vi "FPGA Values View.vi"() -> ()   [LabVIEW 2016, in "M1M3SupportEUI_Views.lvlib"]
uses:
  M1M3SupportEUI_Views.lvlib
  Model/Model.lvclass
  M1M3 Support Events/M1M3 Support Events.lvclass/M1M3 Support Events.ctl
  Typedefs/StateTypes.ctl
  M1M3 Support Events/M1M3 Support Events.lvclass
  Typedefs/M1M3SupportEUI_TypeDefs.lvlib
panel:
  out "Slewing?":string
  out "BroadcastCounter":u8
  out "OuterLoop Time Stamp":timestamp
  out "MRFC 5":u32
  out "MRFC 4":u32
  out "MRFC 3":u32
  out "MRFC 2":u32
  out "MRFC 1":u32
  out "MRBC 5":u32
  out "MRBC 4":u32
  out "MRBC 3":u32
  out "MRBC 2":u32
  out "MRBC 1":u32
  out "MTFC 5":u32
  out "MTFC 4":u32
  out "MTFC 3":u32
  out "MTFC 2":u32
  out "MTFC 1":u32
  out "MTBC 5":u32
  out "MTBC 4":u32
  out "MTBC 3":u32
  out "MTBC 2":u32
  out "MTBC 1":u32
  out "MRDFO 5":string
  out "MRDFO 4":string
  out "MRDFO 3":string
  out "MRDFO 2":string
  out "MRDFO 1":string
  out "MStpBE 5":string
  out "MStpBE 4":string
  out "MStpBE 3":string
  out "MStpBE 2":string
  out "MStpBE 1":string
  out "MStrtBE 5":string
  out "MStrtBE 4":string
  out "MStrtBE 3":string
  out "MStrtBE 2":string
  out "MStrtBE 1":string
  out "MWFRT 5":string
  out "MWFRT 4":string
  out "MWFRT 3":string
  out "MWFRT 2":string
  out "MWFRT 1":string
  out "MII 5":string
  out "MII 4":string
  out "MII 3":string
  out "MII 2":string
  out "MII 1":string
  out "MTIFO1 5":string
  out "MTIFO1 4":string
  out "MTIFO1 3":string
  out "MTIFO1 2":string
  out "MTIFO1":string
  out "FPGA Time Stamp":timestamp
  out "SAL Time Stamp":timestamp
  in  "Model in":refnum<class "Model.lvclass">
  # "FPGA/Outer Loop Data Values"
  # "FPGA"
  # "1"
  # "2"
  # "3"
  # "4"
  # "5"
  # "Modbus TX Internal FIFO Overflow"
  # "Modbus Invalid Instruction"
  # "Modbus Wait For RX Frame Timeout"
  # "Modbus Start Bit Error"
  # "Modbus Stop Bit Error"
  # "Modbus RX Data FIFO Overflow"
  # "Modbus TX Byte Count"
  # "Modbus Tx Frame Count"
  # "Modbus Rx Byte Count"
  # "Modbus Rx Frame Count"
  # "Outer Loop"
  # "Broadcast counter"
  # "Slewing?"
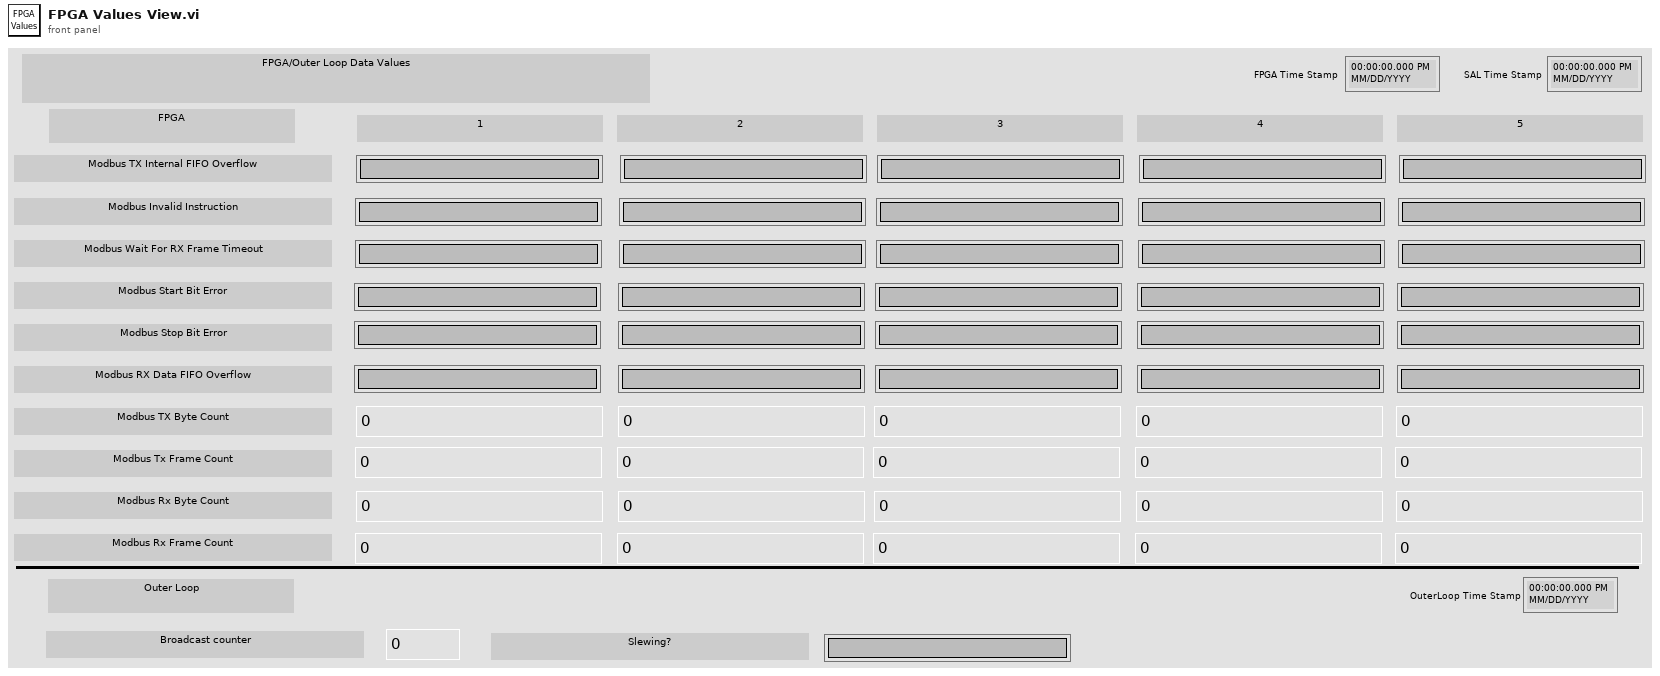
[diagram p1: front panel]
types:
  T1 = typedef "M1M3SupportEUI_TypeDefs.lvlib/M1M3 Support Events.ctl" = cluster{"M1M3 Support State":refnum<user-event>, "Inclinometer  Data":refnum<user-event>, "IMS Data":refnum<user-event>, "FA Data":refnum<user-event>, "FA Status":refnum<user-event>, "SAL Connected":refnum<user-event>, "HP Data":refnum<user-event>, "HP Status":refnum<user-event>, "Accelerometer Data":refnum<user-event>, "FPGA Data":refnum<user-event>, "Inclinometer Data":refnum<user-event>, "MirrorForces Data":refnum<user-event>, "OuterLoop Data":refnum<user-event>, "ErrorCode Event":refnum<user-event>, "InterlockStatus Event":refnum<user-event>, "InterlockWarning Event":refnum<user-event>}
  T2 = typedef "M1M3SupportEUI_TypeDefs.lvlib/StateTypes.ctl" = u32
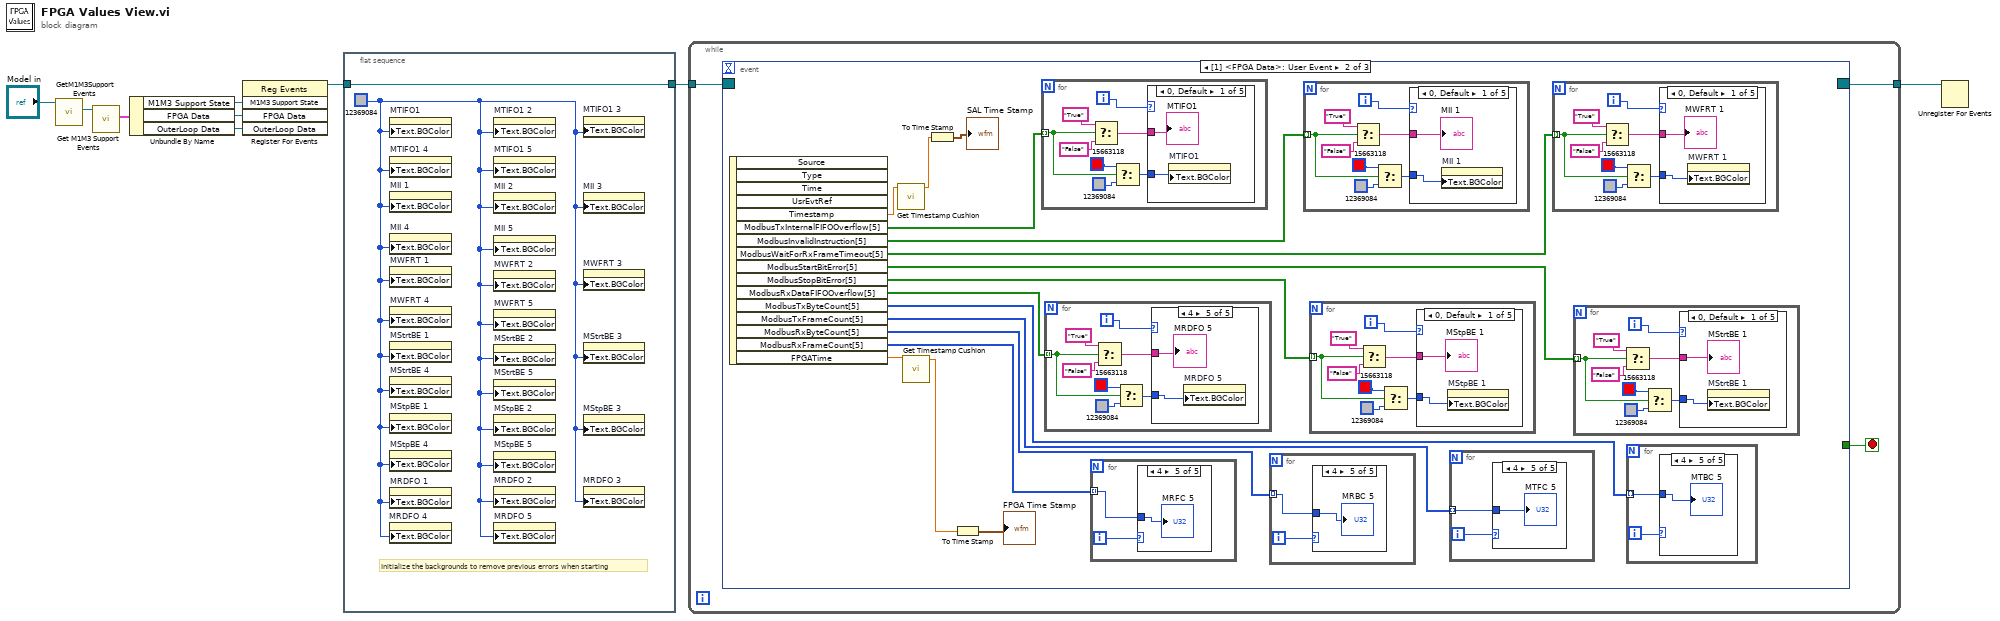
[diagram p0: block diagram]
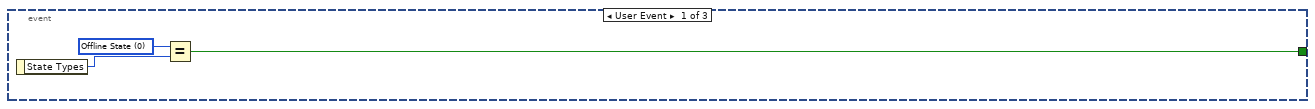
[diagram p2: hidden frame]
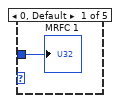
[diagram p3: hidden frame]
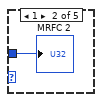
[diagram p4: hidden frame]
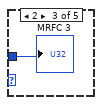
[diagram p5: hidden frame]
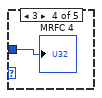
[diagram p6: hidden frame]
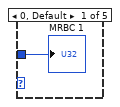
[diagram p7: hidden frame]
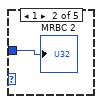
[diagram p8: hidden frame]
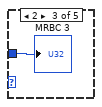
[diagram p9: hidden frame]
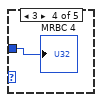
[diagram p10: hidden frame]
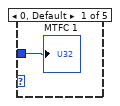
[diagram p11: hidden frame]
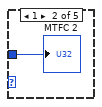
[diagram p12: hidden frame]
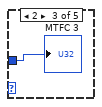
[diagram p13: hidden frame]
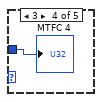
[diagram p14: hidden frame]
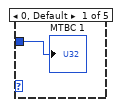
[diagram p15: hidden frame]
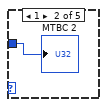
[diagram p16: hidden frame]
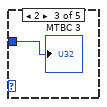
[diagram p17: hidden frame]
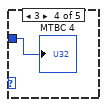
[diagram p18: hidden frame]
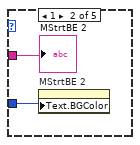
[diagram p19: hidden frame]
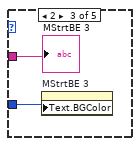
[diagram p20: hidden frame]
diagram:
  n1 = call "GetM1M3SupportEvents.vi"("Model in"="Model in") -> ("M1M3 Support Events out"=w5:refnum<class "M1M3 Support Events.lvclass">)  [unwired: 8 in, 2 out]
  n2 = call "Get M1M3 Support Events.vi"("M1M3 Support Events in"=w5) -> ("M1M3 Support Events"=w6:T1)  [unwired: 9 in, 1 out]
  n3 = Unbundle By Name(w6) -> ("M1M3 Support State"=w8:refnum<user-event>, "FPGA Data"=w9:refnum<user-event>, "OuterLoop Data"=w3:refnum<user-event>)
  n4 = register-events(w8, w9, w3) -> (reference out=w2:refnum<event-registration>)  [unwired: 2 in, 1 out]
  n5 = flat-sequence {
    tunnel: w2 -> [w10]
    tunnel: [w10] -> w1
    frame #0 {
      w11 = u32 12369084
      # "Initialize the backgrounds to remove previous errors when starting"
      n6 = property on="MTIFO1" class="Str"("Text.BGColor"=w11) -> ()  [unwired: 2 in, 2 out]
      n7 = property on="MTIFO1 4" class="Str"("Text.BGColor"=w11) -> ()  [unwired: 2 in, 2 out]
      n8 = property on="MII 1" class="Str"("Text.BGColor"=w11) -> ()  [unwired: 2 in, 2 out]
      n9 = property on="MII 4" class="Str"("Text.BGColor"=w11) -> ()  [unwired: 2 in, 2 out]
      n10 = property on="MWFRT 1" class="Str"("Text.BGColor"=w11) -> ()  [unwired: 2 in, 2 out]
      n11 = property on="MWFRT 4" class="Str"("Text.BGColor"=w11) -> ()  [unwired: 2 in, 2 out]
      n12 = property on="MStrtBE 1" class="Str"("Text.BGColor"=w11) -> ()  [unwired: 2 in, 2 out]
      n13 = property on="MStrtBE 4" class="Str"("Text.BGColor"=w11) -> ()  [unwired: 2 in, 2 out]
      n14 = property on="MStpBE 1" class="Str"("Text.BGColor"=w11) -> ()  [unwired: 2 in, 2 out]
      n15 = property on="MStpBE 4" class="Str"("Text.BGColor"=w11) -> ()  [unwired: 2 in, 2 out]
      n16 = property on="MRDFO 1" class="Str"("Text.BGColor"=w11) -> ()  [unwired: 2 in, 2 out]
      n17 = property on="MRDFO 4" class="Str"("Text.BGColor"=w11) -> ()  [unwired: 2 in, 2 out]
      n18 = property on="MTIFO1 2" class="Str"("Text.BGColor"=w11) -> ()  [unwired: 2 in, 2 out]
      n19 = property on="MTIFO1 5" class="Str"("Text.BGColor"=w11) -> ()  [unwired: 2 in, 2 out]
      n20 = property on="MII 2" class="Str"("Text.BGColor"=w11) -> ()  [unwired: 2 in, 2 out]
      n21 = property on="MII 5" class="Str"("Text.BGColor"=w11) -> ()  [unwired: 2 in, 2 out]
      n22 = property on="MWFRT 2" class="Str"("Text.BGColor"=w11) -> ()  [unwired: 2 in, 2 out]
      n23 = property on="MWFRT 5" class="Str"("Text.BGColor"=w11) -> ()  [unwired: 2 in, 2 out]
      n24 = property on="MStrtBE 2" class="Str"("Text.BGColor"=w11) -> ()  [unwired: 2 in, 2 out]
      n25 = property on="MStrtBE 5" class="Str"("Text.BGColor"=w11) -> ()  [unwired: 2 in, 2 out]
      n26 = property on="MStpBE 2" class="Str"("Text.BGColor"=w11) -> ()  [unwired: 2 in, 2 out]
      n27 = property on="MStpBE 5" class="Str"("Text.BGColor"=w11) -> ()  [unwired: 2 in, 2 out]
      n28 = property on="MRDFO 2" class="Str"("Text.BGColor"=w11) -> ()  [unwired: 2 in, 2 out]
      n29 = property on="MRDFO 5" class="Str"("Text.BGColor"=w11) -> ()  [unwired: 2 in, 2 out]
      n30 = property on="MTIFO1 3" class="Str"("Text.BGColor"=w11) -> ()  [unwired: 2 in, 2 out]
      n31 = property on="MII 3" class="Str"("Text.BGColor"=w11) -> ()  [unwired: 2 in, 2 out]
      n32 = property on="MWFRT 3" class="Str"("Text.BGColor"=w11) -> ()  [unwired: 2 in, 2 out]
      n33 = property on="MStrtBE 3" class="Str"("Text.BGColor"=w11) -> ()  [unwired: 2 in, 2 out]
      n34 = property on="MStpBE 3" class="Str"("Text.BGColor"=w11) -> ()  [unwired: 2 in, 2 out]
      n35 = property on="MRDFO 3" class="Str"("Text.BGColor"=w11) -> ()  [unwired: 2 in, 2 out]
    }
  }
  n36 = while {
    tunnel: w1 -> [w14]
    tunnel: [w12] -> w4
    stop <- w13 stop-if-true
    n37 = event shown="[1] <FPGA Data>: User Event" {
      selector: w14 -> [_ _ _]
      dyn-events: [_ _ _] -> w12
      timeout: _ -> [_ _ _]
      tunnel: [w15 _ _] -> w13
      event User Event {
        w16 = T2 0 items=["Offline State"=0, "Fault State"=4294967295, "Standby State"=16777216, "Disabled State"=33554432, "Enabled State"=50331648, "Parked State"=50331649, "Raising State"=50331650, "Active State"=50331651, "Lowering State"=50331652, "Engineering State"=50397184, "Parked Engineering State"=50397185, "Raising Engineering State"=50397186, "Active Engineering State"=50397187, "Lowering Engineering State"=50397188] ("x")
        n38 = event-data() -> ("State Types"=w17:T2)  [unwired: 1 in]
        n39 = Equal?(x=w16, y=w17) -> (x = y?=w15:bool)
      }
      event User Event {
        n40 = event-data() -> ("Timestamp"=w19:dbl, "ModbusTxInternalFIFOOverflow[5]"=w33:bool[], "ModbusInvalidInstruction[5]"=w32:bool[], "ModbusWaitForRxFrameTimeout[5]"=w31:bool[], "ModbusStartBitError[5]"=w28:bool[], "ModbusStopBitError[5]"=w29:bool[], "ModbusRxDataFIFOOverflow[5]"=w30:bool[], "ModbusTxByteCount[5]"=w27:u32[], "ModbusTxFrameCount[5]"=w26:u32[], "ModbusRxByteCount[5]"=w25:u32[], "ModbusRxFrameCount[5]"=w24:u32[], "FPGATime"=w21:dbl)  [unwired: 1 in, 4 out]
        n41 = call "Get Timestamp Cushion.vi"("DoubleTimestampRepresentation"=w19) -> ("TimestampCushion"=w18:dbl)  [unwired: 10 in]
        n42 = call "Get Timestamp Cushion.vi"("DoubleTimestampRepresentation"=w21) -> ("TimestampCushion"=w20:dbl)  [unwired: 10 in]
        n43 = To Time Stamp(1:w18) -> (0:→"SAL Time Stamp":timestamp)
        n44 = To Time Stamp(1:w20) -> (0:→"FPGA Time Stamp":timestamp)
        n45 = for {
          tunnel: w33 -> [w153] mode=indexing
          i -> [w157]
          n46 = Select(t="True", s=w153, f="False") -> (s? t:f=w156:string)
          n47 = Select(t=u32 15663118, s=w153, f=u32 12369084) -> (s? t:f=w152:u32)
          n48 = case shown="0, Default" w157 {
            tunnel: w156 -> [w161 w163 w165 w167 w169]
            tunnel: w152 -> [w160 w162 w164 w166 w168]
            frame 0, Default {
              n49 = property on="MTIFO1" class="Str"("Text.BGColor"=w160) -> ()  [unwired: 2 in, 2 out]
              "MTIFO1" <- w161
            }
            frame 1 {
              n50 = property on="MTIFO1 2" class="Str"("Text.BGColor"=w162) -> ()  [unwired: 2 in, 2 out]
              "MTIFO1 2" <- w163
            }
            frame 2 {
              n51 = property on="MTIFO1 3" class="Str"("Text.BGColor"=w164) -> ()  [unwired: 2 in, 2 out]
              "MTIFO1 3" <- w165
            }
            frame 3 {
              n52 = property on="MTIFO1 4" class="Str"("Text.BGColor"=w166) -> ()  [unwired: 2 in, 2 out]
              "MTIFO1 4" <- w167
            }
            frame 4 {
              n53 = property on="MTIFO1 5" class="Str"("Text.BGColor"=w168) -> ()  [unwired: 2 in, 2 out]
              "MTIFO1 5" <- w169
            }
          }
        }
        n54 = for {
          tunnel: w30 -> [w99] mode=indexing
          i -> [w103]
          n55 = Select(t="True", s=w99, f="False") -> (s? t:f=w102:string)
          n56 = Select(t=u32 15663118, s=w99, f=u32 12369084) -> (s? t:f=w98:u32)
          n57 = case shown="4" w103 {
            tunnel: w102 -> [w107 w109 w111 w113 w115]
            tunnel: w98 -> [w106 w108 w110 w112 w114]
            frame 0, Default {
              n58 = property on="MRDFO 1" class="Str"("Text.BGColor"=w106) -> ()  [unwired: 2 in, 2 out]
              "MRDFO 1" <- w107
            }
            frame 1 {
              n59 = property on="MRDFO 2" class="Str"("Text.BGColor"=w108) -> ()  [unwired: 2 in, 2 out]
              "MRDFO 2" <- w109
            }
            frame 2 {
              n60 = property on="MRDFO 3" class="Str"("Text.BGColor"=w110) -> ()  [unwired: 2 in, 2 out]
              "MRDFO 3" <- w111
            }
            frame 3 {
              n61 = property on="MRDFO 4" class="Str"("Text.BGColor"=w112) -> ()  [unwired: 2 in, 2 out]
              "MRDFO 4" <- w113
            }
            frame 4 {
              n62 = property on="MRDFO 5" class="Str"("Text.BGColor"=w114) -> ()  [unwired: 2 in, 2 out]
              "MRDFO 5" <- w115
            }
          }
        }
        n63 = for {
          tunnel: w24 -> [w34] mode=indexing
          i -> [w35]
          n64 = case shown="4" w35 {
            tunnel: w34 -> [w36 w37 w38 w39 w40]
            frame 0, Default {
              "MRFC 1" <- w36
            }
            frame 1 {
              "MRFC 2" <- w37
            }
            frame 2 {
              "MRFC 3" <- w38
            }
            frame 3 {
              "MRFC 4" <- w39
            }
            frame 4 {
              "MRFC 5" <- w40
            }
          }
        }
        n65 = for {
          tunnel: w25 -> [w41] mode=indexing
          i -> [w42]
          n66 = case shown="4" w42 {
            tunnel: w41 -> [w43 w44 w45 w46 w47]
            frame 0, Default {
              "MRBC 1" <- w43
            }
            frame 1 {
              "MRBC 2" <- w44
            }
            frame 2 {
              "MRBC 3" <- w45
            }
            frame 3 {
              "MRBC 4" <- w46
            }
            frame 4 {
              "MRBC 5" <- w47
            }
          }
        }
        n67 = for {
          tunnel: w32 -> [w135] mode=indexing
          i -> [w139]
          n68 = Select(t="True", s=w135, f="False") -> (s? t:f=w138:string)
          n69 = Select(t=u32 15663118, s=w135, f=u32 12369084) -> (s? t:f=w134:u32)
          n70 = case shown="0, Default" w139 {
            tunnel: w138 -> [w143 w145 w147 w149 w151]
            tunnel: w134 -> [w142 w144 w146 w148 w150]
            frame 0, Default {
              n71 = property on="MII 1" class="Str"("Text.BGColor"=w142) -> ()  [unwired: 2 in, 2 out]
              "MII 1" <- w143
            }
            frame 1 {
              n72 = property on="MII 2" class="Str"("Text.BGColor"=w144) -> ()  [unwired: 2 in, 2 out]
              "MII 2" <- w145
            }
            frame 2 {
              n73 = property on="MII 3" class="Str"("Text.BGColor"=w146) -> ()  [unwired: 2 in, 2 out]
              "MII 3" <- w147
            }
            frame 3 {
              n74 = property on="MII 4" class="Str"("Text.BGColor"=w148) -> ()  [unwired: 2 in, 2 out]
              "MII 4" <- w149
            }
            frame 4 {
              n75 = property on="MII 5" class="Str"("Text.BGColor"=w150) -> ()  [unwired: 2 in, 2 out]
              "MII 5" <- w151
            }
          }
        }
        n76 = for {
          tunnel: w29 -> [w81] mode=indexing
          i -> [w85]
          n77 = Select(t="True", s=w81, f="False") -> (s? t:f=w84:string)
          n78 = Select(t=u32 15663118, s=w81, f=u32 12369084) -> (s? t:f=w80:u32)
          n79 = case shown="0, Default" w85 {
            tunnel: w84 -> [w89 w91 w93 w95 w97]
            tunnel: w80 -> [w88 w90 w92 w94 w96]
            frame 0, Default {
              n80 = property on="MStpBE 1" class="Str"("Text.BGColor"=w88) -> ()  [unwired: 2 in, 2 out]
              "MStpBE 1" <- w89
            }
            frame 1 {
              n81 = property on="MStpBE 2" class="Str"("Text.BGColor"=w90) -> ()  [unwired: 2 in, 2 out]
              "MStpBE 2" <- w91
            }
            frame 2 {
              n82 = property on="MStpBE 3" class="Str"("Text.BGColor"=w92) -> ()  [unwired: 2 in, 2 out]
              "MStpBE 3" <- w93
            }
            frame 3 {
              n83 = property on="MStpBE 4" class="Str"("Text.BGColor"=w94) -> ()  [unwired: 2 in, 2 out]
              "MStpBE 4" <- w95
            }
            frame 4 {
              n84 = property on="MStpBE 5" class="Str"("Text.BGColor"=w96) -> ()  [unwired: 2 in, 2 out]
              "MStpBE 5" <- w97
            }
          }
        }
        n85 = for {
          tunnel: w26 -> [w48] mode=indexing
          i -> [w49]
          n86 = case shown="4" w49 {
            tunnel: w48 -> [w50 w51 w52 w53 w54]
            frame 0, Default {
              "MTFC 1" <- w50
            }
            frame 1 {
              "MTFC 2" <- w51
            }
            frame 2 {
              "MTFC 3" <- w52
            }
            frame 3 {
              "MTFC 4" <- w53
            }
            frame 4 {
              "MTFC 5" <- w54
            }
          }
        }
        n87 = for {
          tunnel: w31 -> [w117] mode=indexing
          i -> [w121]
          n88 = Select(t="True", s=w117, f="False") -> (s? t:f=w120:string)
          n89 = Select(t=u32 15663118, s=w117, f=u32 12369084) -> (s? t:f=w116:u32)
          n90 = case shown="0, Default" w121 {
            tunnel: w120 -> [w125 w127 w129 w131 w133]
            tunnel: w116 -> [w124 w126 w128 w130 w132]
            frame 0, Default {
              n91 = property on="MWFRT 1" class="Str"("Text.BGColor"=w124) -> ()  [unwired: 2 in, 2 out]
              "MWFRT 1" <- w125
            }
            frame 1 {
              n92 = property on="MWFRT 2" class="Str"("Text.BGColor"=w126) -> ()  [unwired: 2 in, 2 out]
              "MWFRT 2" <- w127
            }
            frame 2 {
              n93 = property on="MWFRT 3" class="Str"("Text.BGColor"=w128) -> ()  [unwired: 2 in, 2 out]
              "MWFRT 3" <- w129
            }
            frame 3 {
              n94 = property on="MWFRT 4" class="Str"("Text.BGColor"=w130) -> ()  [unwired: 2 in, 2 out]
              "MWFRT 4" <- w131
            }
            frame 4 {
              n95 = property on="MWFRT 5" class="Str"("Text.BGColor"=w132) -> ()  [unwired: 2 in, 2 out]
              "MWFRT 5" <- w133
            }
          }
        }
        n96 = for {
          tunnel: w28 -> [w63] mode=indexing
          i -> [w67]
          n97 = Select(t="True", s=w63, f="False") -> (s? t:f=w66:string)
          n98 = Select(t=u32 15663118, s=w63, f=u32 12369084) -> (s? t:f=w62:u32)
          n99 = case shown="0, Default" w67 {
            tunnel: w66 -> [w71 w73 w75 w77 w79]
            tunnel: w62 -> [w70 w72 w74 w76 w78]
            frame 0, Default {
              n100 = property on="MStrtBE 1" class="Str"("Text.BGColor"=w70) -> ()  [unwired: 2 in, 2 out]
              "MStrtBE 1" <- w71
            }
            frame 1 {
              n101 = property on="MStrtBE 2" class="Str"("Text.BGColor"=w72) -> ()  [unwired: 2 in, 2 out]
              "MStrtBE 2" <- w73
            }
            frame 2 {
              n102 = property on="MStrtBE 3" class="Str"("Text.BGColor"=w74) -> ()  [unwired: 2 in, 2 out]
              "MStrtBE 3" <- w75
            }
            frame 3 {
              n103 = property on="MStrtBE 4" class="Str"("Text.BGColor"=w76) -> ()  [unwired: 2 in, 2 out]
              "MStrtBE 4" <- w77
            }
            frame 4 {
              n104 = property on="MStrtBE 5" class="Str"("Text.BGColor"=w78) -> ()  [unwired: 2 in, 2 out]
              "MStrtBE 5" <- w79
            }
          }
        }
        n105 = for {
          tunnel: w27 -> [w55] mode=indexing
          i -> [w56]
          n106 = case shown="4" w56 {
            tunnel: w55 -> [w57 w58 w59 w60 w61]
            frame 0, Default {
              "MTBC 1" <- w57
            }
            frame 1 {
              "MTBC 2" <- w58
            }
            frame 2 {
              "MTBC 3" <- w59
            }
            frame 3 {
              "MTBC 4" <- w60
            }
            frame 4 {
              "MTBC 5" <- w61
            }
          }
        }
      }
      event User Event {
        n107 = event-data() -> ("Timestamp"=w177:dbl, "BroadcastCounter"=→"BroadcastCounter":u8, "SlewFlag"=w172:bool)  [unwired: 1 in, 4 out]
        n108 = call "Get Timestamp Cushion.vi"("DoubleTimestampRepresentation"=w177) -> ("TimestampCushion"=w176:dbl)  [unwired: 10 in]
        n109 = Select(t="True", s=w172, f="False") -> (s? t:f=→"Slewing?":string)
        n110 = To Time Stamp(1:w176) -> (0:→"OuterLoop Time Stamp":timestamp)
      }
    }
  }
  n111 = Unregister For Events(event registration refnum=w4) -> ()  [unwired: 1 in, 1 out]
